vi "Check Is Installed Library.vi"(8 "error in (no error)":errorcluster, 11 "Item Path":path) -> (0 "error out":errorcluster, 3 "Is Installed Library?":bool)   [LabVIEW 2015, in "Add License to VI Documentation.lvlib"]
uses:
  Add License to VI Documentation.lvlib
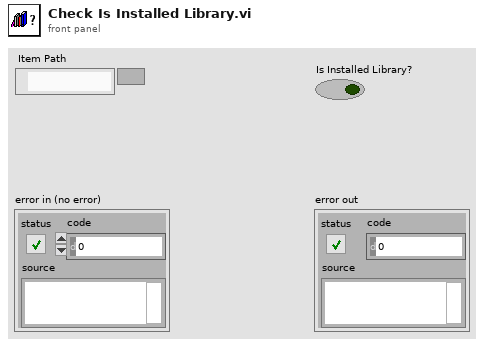
[diagram p1: front panel]
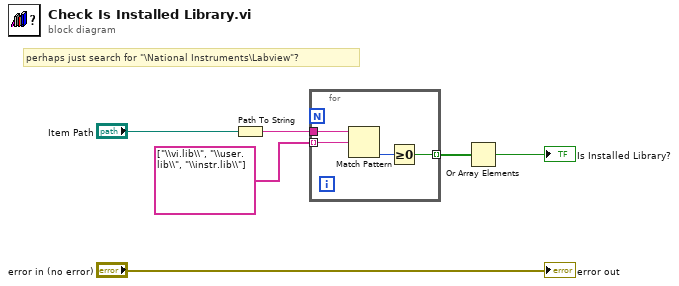
[diagram p0: block diagram]
diagram:
  # "perhaps just search for \"\\National Instruments\\Labview\"?"
  n1 = Path To String(path="Item Path") -> (string=w4:string)
  n2 = for {
    tunnel: w4 -> [w10]
    tunnel: string[] ["\\vi.lib\\", "\\user.lib\\", "\\instr.lib\\"] ("regular expression") -> [w9] mode=indexing
    tunnel: [w7] -> w2 mode=indexing
    n3 = Match Pattern(string=w10, regular expression=w9) -> (offset past match=w8:i32)  [unwired: 1 in, 3 out]
    n4 = Greater Or Equal To 0?(x=w8) -> (x >= 0?=w7:bool)
  }
  n5 = Or Array Elements(Boolean array=w2) -> (logical OR=→"Is Installed Library?":bool)
  "error out" <- "error in (no error)"
